vi "diff CALC.vi"() -> ()   [LabVIEW 2016]
uses:
  <userlib>/_MGI/1D Array/MGI Calculate Array Differences/MGI Calculate Array Differences (DBL[]).vi
panel:
  out "y(i)=x(i)-x(i-1)":dbl[](array[numeric]) format="%.2f"
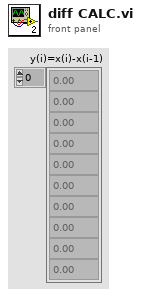
[diagram p1: front panel]
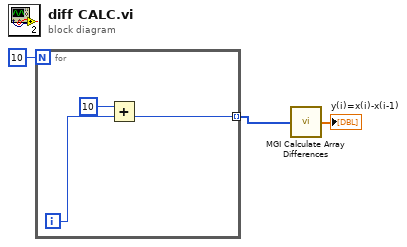
[diagram p0: block diagram]
diagram:
  n1 = for {
    N: 10 -> [_]
    tunnel: [w5] -> w2 mode=indexing
    i -> [w6]
    n2 = Add(x=10, y=w6) -> (x+y=w5:i32)
  }
  n3 = call-poly <userlib>:"MGI Calculate Array Differences.vi"("x(i)"=w2) -> ("y(i)=x(i)-x(i-1)"=→"y(i)=x(i)-x(i-1)":dbl[])  [unwired: 1 in]
